vi "DMA_ReadUI.vi"() -> ()   [LabVIEW 2014, in "DMA_Read.lvclass"]
doc: "Template for creating new user-interface VIs for inherited classes."
uses:
  DMA_Read.lvclass
  <vilib>/NI/AMC/Message Queue.ctl
  <vilib>/NI/AMC/Message.ctl
  <vilib>/NI/Tools/Keyed Array/KeyedArray.ctl
  xCE/xceTreeObj/xceTreeObj.lvclass
  <vilib>/NI/AMC/Read Termination Message.vi
  <vilib>/NI/AMC/Create Single Message.vi
  <vilib>/NI/AMC/Update Message Routing Info.vi
  <vilib>/NI/AMC/Globals.vi
  <vilib>/NI/AMC/Send Message.vi
  <vilib>/NI/AMC/AMC.lvlib
  xCE/xceNode/xceNode.lvclass
  <vilib>/NI/Tools/Keyed Array/Tools_KeyedArray.lvlib
panel:
  out "Number of Packets":i32
  in  "DataNode*":refnum<data-value>
  in  "AMC*":T1
  in  "Exit":bool
  # "(Does NOT Include the Void Type Packets)"
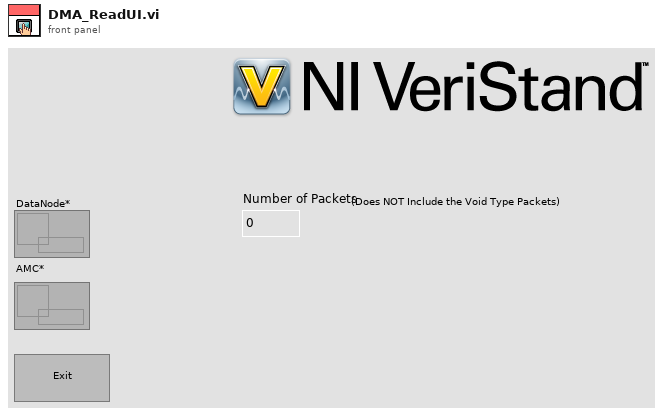
[diagram p1: front panel]
types:
  T1 = typedef "AMC.lvlib/Message Queue.ctl" = refnum<queue>
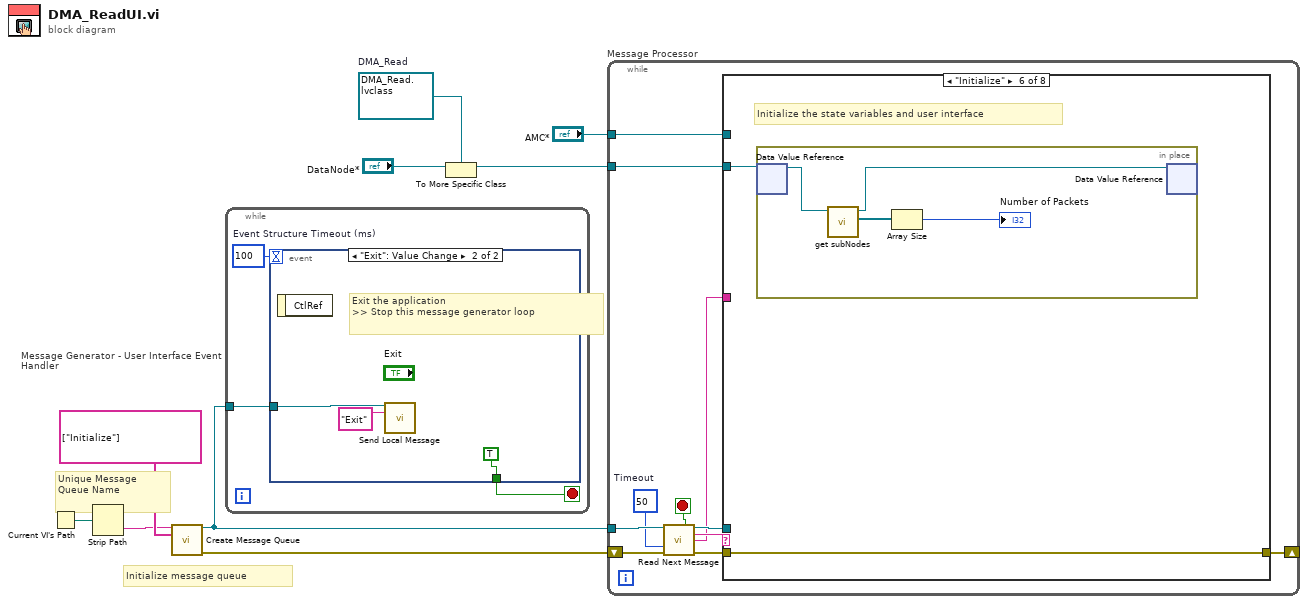
[diagram p0: block diagram]
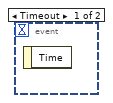
[diagram p2: hidden frame]
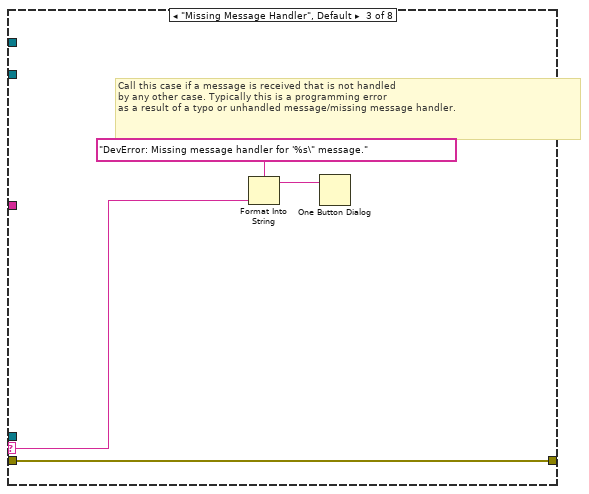
[diagram p5: hidden frame]
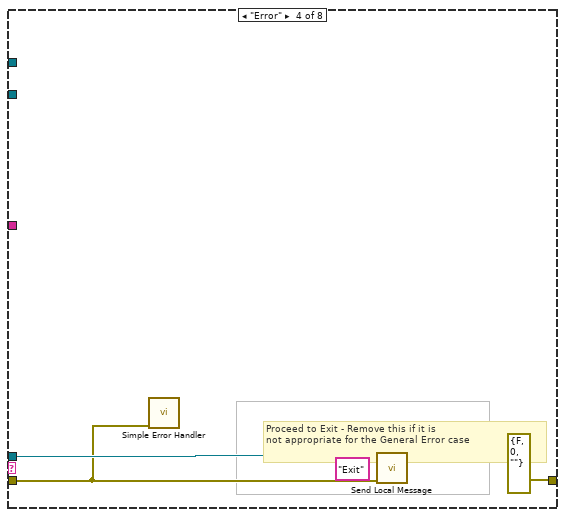
[diagram p6: hidden frame]
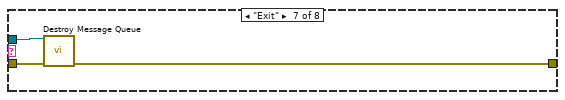
[diagram p8: hidden frame]
diagram:
  w1 = refnum<data-value> refnum  # DMA_Read
  # "Initialize message queue"
  # "Unique Message\nQueue Name"
  n1 = Current VI's Path() -> (path=w5:path)
  n2 = Strip Path(path=w5) -> (name=w8:string)  [unwired: 1 out]
  n3 = call <vilib>:"Create Message Queue.vi"("message queue name"=w8, "initial message names"=string[] ["Initialize"]) -> ("message queue out"=w7:T1, "error out"=w6:errorcluster)  [unwired: 12 in]
  n4 = while "Message Generator - User Interface Event Handler" {
    tunnel: w7 -> [w10]
    stop <- w11 stop-if-true
    w12 = 100  # Event Structure Timeout (ms)
    n5 = event shown="[1] \"Exit\": Value Change" {
      selector: _ -> [_ _]
      dyn-events: _ -> [_ _]
      timeout: w12 -> [_ _]
      tunnel: [_ TRUE ("Discard?")] -> w11
      tunnel: w10 -> [_ w13]
      event Timeout {
        n6 = event-data() -> ()  [unwired: 2 out]
      }
      event "Exit": Value Change {
        # "Exit the application\n>> Stop this message generator loop"
        n7 = event-data() -> ()  [unwired: 2 out]
        n8 = call <vilib>:"Send Local Message.vi"("message queue in"=w13, "message name"="Exit") -> ()  [unwired: 11 in, 3 out]
      }
    }
  }
  n9 = To More Specific Class(target class=w1, reference="DataNode*") -> (specific class reference=w2:refnum<data-value>)  [unwired: 1 in, 1 out]
  n10 = while "Message Processor" {
    shift-left: w6 -> [w22]
    shift-right: [w26] -> _
    tunnel: w7 -> [w23]
    tunnel: "AMC*" -> [w17]
    tunnel: w2 -> [w16]
    stop <- w25 stop-if-true
    w20 = 50  # Timeout
    n11 = call <vilib>:"Read Next Message.vi"("message queue in"=w23, "timeout (1 ms)"=w20, "error in"=w22) -> ("exit process?"=w25:bool, "message queue out"=w24:T1, "message name"=w19:string, "message value"=w18:string, "error out"=w21:errorcluster)  [unwired: 5 in, 3 out]
    n12 = case shown="\"Initialize\"" w19 {
      selector: w19 -> [_ _ w31 _ _ _ _ _]
      tunnel: w24 -> [_ _ _ w35 _ _ w45 _]
      tunnel: w21 -> [w27 w28 w32 w33 w37 w39 w46 w47]
      tunnel: [w27 w28 w32 errorcluster {"status"=FALSE, "code"=0, "source"=""} ("error out") w37 w39 w44 w47] -> w26
      tunnel: w18 -> [_ _ _ _ _ _ _ _]
      tunnel: w17 -> [_ _ _ _ _ _ _ _]
      tunnel: w16 -> [_ _ _ _ _ w38 _ _]
      frame "---------- Framework Operations ----------" {
        # "Dummy case to add a seperator in the Case Structure menu"
      }
      frame "", "Idle" {
      }
      frame "Missing Message Handler", Default {
        # "Call this case if a message is received that is not handled \nby any other case. Typically this is a programming error\nas a result of a typo or unhandled message/missing message handler."
        n13 = Format Into String(format string="DevError: Missing message handler for '%s\" message." ("message"), w31) -> (resulting string=w29:string)  [unwired: 2 in, 1 out]
        n14 = One Button Dialog(message=w29) -> ()  [unwired: 2 out]
      }
      frame "Error" {
        # "Proceed to Exit - Remove this if it is\nnot appropriate for the General Error case"
        n15 = call <vilib>:"Simple Error Handler.vi"("error in (no error)"=w33) -> ()  [unwired: 1 in, 8 out]
        n16 = call <vilib>:"Send Local Message.vi"("message queue in"=w35, "message name"="Exit", "error in"=w33) -> ()  [unwired: 10 in, 3 out]
      }
      frame "---------- Generic Operations ----------" {
        # "Dummy case to add a seperator in the Case Structure menu"
      }
      frame "Initialize" {
        # "Initialize the state variables and user interface"
        n17 = in-place {
          n18 = in-place-dvr #1(w38) -> (w43:refnum<class "DMA_Read.lvclass">)  [unwired: 1 out]
          n19 = call "get subNodes.vi"("xceNode in"=w43) -> ("subNodes[]*"=w42:refnum<data-value>[], "xceNode out"=w41:refnum<class "DMA_Read.lvclass">)  [unwired: 8 in, 1 out]
          n20 = Array Size(array=w42) -> (size(s)=→"Number of Packets":i32)
          n21 = in-place-dvr #1(w41) -> ()  [unwired: 2 out]
        }
      }
      frame "Exit" {
        n22 = call <vilib>:"Destroy Message Queue.vi"("message queue in"=w45, "error in"=w46) -> ("error out"=w44:errorcluster)  [unwired: 11 in, 2 out]
      }
      frame "---------- Application Operations ----------" {
        # "Dummy case to add a seperator in the Case Structure menu"
      }
    }
  }
